vi "IIR Cascade Filter with I.C. PtByPt.vi"(0 "x":dbl format="%0.2f", 1 "IIR Filter Cluster":T1, 3 "Initial Condition":dbl[](array[numeric]), 4 "initialize":bool) -> (5 "Filtered x":dbl format="%0.2f", 6 "Final Condition":dbl[](array[numeric]), 7 "error":i32)   [LabVIEW 2020, in "NI_PtbyPt.lvlib"]
doc: "Filters <B>x</B> using the cascade form of the IIR filter specified by the <B>IIR Filter Cluster</B>."
uses:
  <vilib>/ptbypt/NI_PtbyPt.lvlib
  <vilib>/Analysis/baseanly.llb/IIR Cascade Filter (DBL).vi
  <vilib>/Analysis/NI_AALBase.lvlib
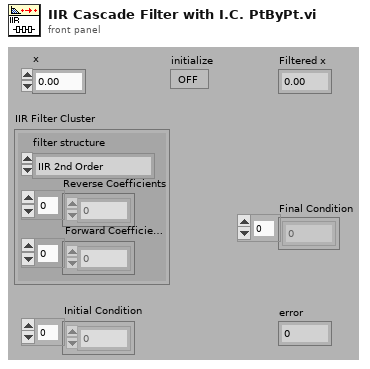
[diagram p1: front panel]
types:
  T1 = cluster{"filter structure":enum32{"IIR 2nd Order", "IIR 4th Order"}, "Reverse Coefficients":dbl[], "Forward Coefficients":dbl[]}
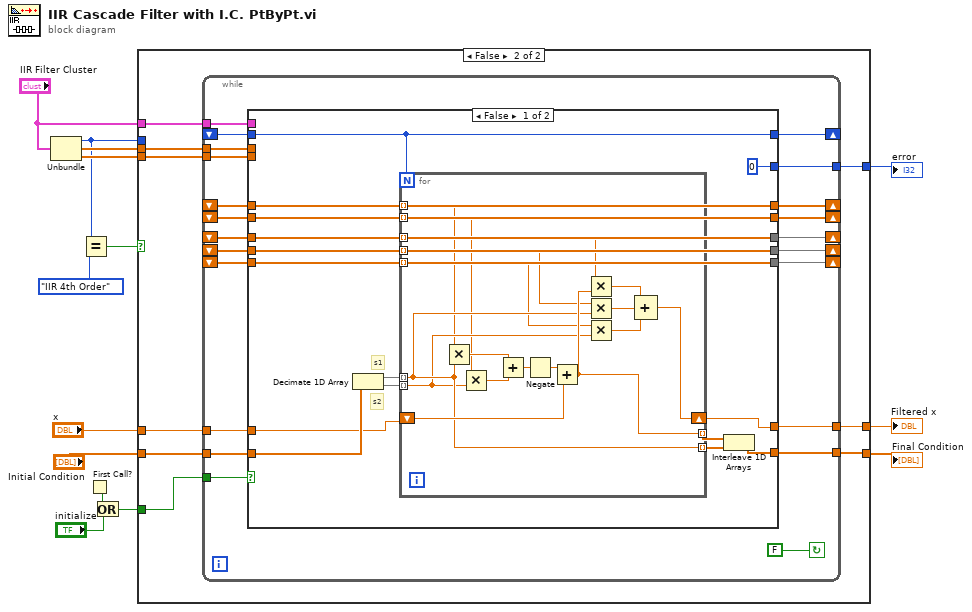
[diagram p0: block diagram]
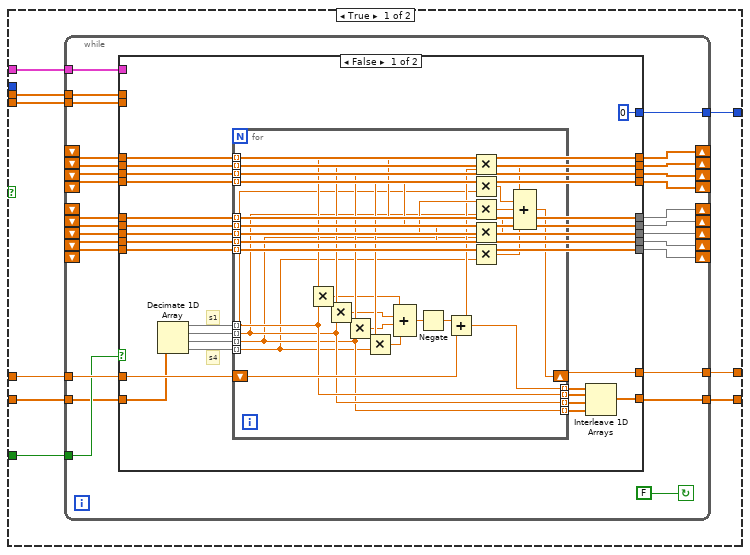
[diagram p2: hidden frame]
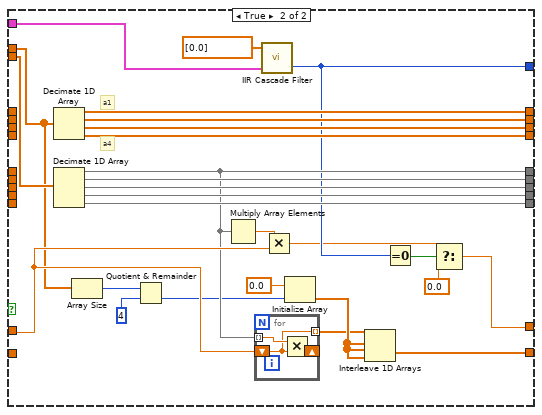
[diagram p3: hidden frame]
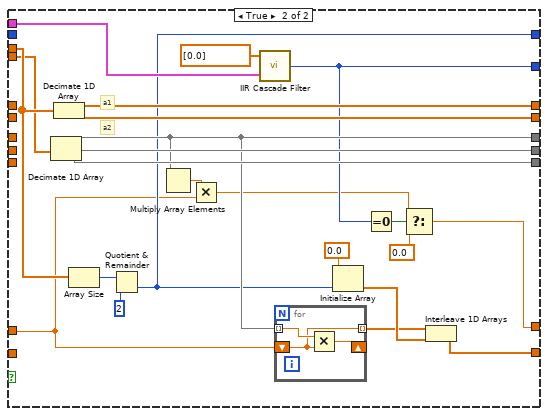
[diagram p4: hidden frame]
diagram:
  n1 = Unbundle("IIR Filter Cluster") -> ("filter structure"=w11:enum32{"IIR 2nd Order", "IIR 4th Order"}, "Reverse Coefficients"=w12:dbl[], "Forward Coefficients"=w13:dbl[])
  n2 = Equal?(x=w11, y=enum32{"IIR 2nd Order", "IIR 4th Order"}."IIR 4th Order") -> (x = y?=w9:bool)
  n3 = First Call?() -> (First Call?: T/F=w6:bool)
  n4 = Or(x=w6, y="initialize") -> (x .or. y?=w7:bool)
  n5 = case shown="False" w9 {
    tunnel: "x" -> [w22 w138]
    tunnel: w13 -> [w20 w136]
    tunnel: w11 -> [_ _]
    tunnel: w12 -> [w21 w137]
    tunnel: [w19 w135] -> w8
    tunnel: w7 -> [w23 w139]
    tunnel: "IIR Filter Cluster" -> [w18 w134]
    tunnel: [w17 w133] -> w4
    tunnel: "Initial Condition" -> [w15 w131]
    tunnel: [w16 w132] -> w2
    frame True {
      n6 = while {
        tunnel: w15 -> [w24]
        tunnel: [w25] -> w16
        tunnel: [w27] -> w17
        tunnel: w18 -> [w28]
        tunnel: [w30] -> w19
        shift-left: _ -> [w31]
        shift-right: [w32] -> _
        shift-left: _ -> [w33]
        shift-right: [w35] -> _
        shift-left: _ -> [w34]
        shift-right: [w36] -> _
        shift-left: _ -> [w37]
        shift-right: [w38] -> _
        tunnel: w22 -> [w39]
        tunnel: w21 -> [w40]
        shift-left: _ -> [w41]
        shift-right: [w43] -> _
        shift-left: _ -> [w42]
        shift-right: [w44] -> _
        shift-left: _ -> [w46]
        shift-right: [w49] -> _
        shift-left: _ -> [w45]
        shift-right: [w48] -> _
        shift-left: _ -> [w47]
        shift-right: [w50] -> _
        tunnel: w20 -> [w51]
        tunnel: w23 -> [w26]
        stop <- FALSE continue-if-true
        n7 = case shown="False" w26 {
          tunnel: w51 -> [_ w116]
          tunnel: [w68 w123] -> w50
          tunnel: [w67 w122] -> w49
          tunnel: [w66 w121] -> w48
          tunnel: w47 -> [w68 _]
          tunnel: w46 -> [w67 _]
          tunnel: w45 -> [w66 _]
          tunnel: [w71 w125] -> w44
          tunnel: [w70 w124] -> w43
          tunnel: w42 -> [w71 _]
          tunnel: w41 -> [w70 _]
          tunnel: w40 -> [_ w104]
          tunnel: w39 -> [w60 w114]
          tunnel: [w72 w126] -> w38
          tunnel: w37 -> [w72 _]
          tunnel: [w69 w113] -> w36
          tunnel: [w65 w120] -> w35
          tunnel: w34 -> [w69 _]
          tunnel: w33 -> [w65 _]
          tunnel: [w73 w127] -> w32
          tunnel: w31 -> [w73 _]
          tunnel: [w58 w106] -> w30
          tunnel: w24 -> [w59 _]
          tunnel: [w53 w115] -> w25
          tunnel: w28 -> [_ w111]
          tunnel: [0 ("error") w109] -> w27
          frame False {
            # "s4"
            # "s1"
            n8 = Decimate 1D Array(w59) -> (w64:dbl[], w63:dbl[], w62:dbl[], w61:dbl[])
            n9 = for {
              tunnel: w71 -> [w98] mode=indexing
              tunnel: w70 -> [w97] mode=indexing
              tunnel: w68 -> [w89] mode=indexing
              tunnel: w67 -> [w88] mode=indexing
              tunnel: w66 -> [w87] mode=indexing
              tunnel: w72 -> [w99] mode=indexing
              tunnel: w65 -> [w86] mode=indexing
              tunnel: w73 -> [w100] mode=indexing
              tunnel: w69 -> [w90] mode=indexing
              tunnel: w64 -> [w77] mode=indexing
              tunnel: w63 -> [w76] mode=indexing
              tunnel: w62 -> [w75] mode=indexing
              tunnel: w61 -> [w74] mode=indexing
              tunnel: [w78] -> w57 mode=indexing
              tunnel: [w75] -> w54 mode=indexing
              tunnel: [w76] -> w55 mode=indexing
              tunnel: [w77] -> w56 mode=indexing
              shift-right: [w79] -> w58
              shift-left: w60 -> [w80]
              n10 = Multiply(x=w100, y=w77) -> (x*y=w96:dbl)
              n11 = Multiply(x=w99, y=w76) -> (x*y=w95:dbl)
              n12 = Multiply(x=w98, y=w75) -> (x*y=w94:dbl)
              n13 = Multiply(x=w97, y=w74) -> (x*y=w93:dbl)
              n14 = Compound Arithmetic op=ADD(w96, w95, w94, w93) -> (w92:dbl)
              n15 = Negate(x=w92) -> (-x=w91:dbl)
              n16 = Add(x=w91, y=w80) -> (x+y=w78:dbl)
              n17 = Multiply(x=w90, y=w78) -> (x*y=w85:dbl)
              n18 = Multiply(x=w89, y=w77) -> (x*y=w84:dbl)
              n19 = Multiply(x=w88, y=w76) -> (x*y=w83:dbl)
              n20 = Multiply(x=w87, y=w75) -> (x*y=w82:dbl)
              n21 = Multiply(x=w86, y=w74) -> (x*y=w81:dbl)
              n22 = Compound Arithmetic op=ADD(w85, w84, w83, w82, w81) -> (w79:dbl)
            }
            n23 = Interleave 1D Arrays(w57, w56, w55, w54) -> (w53:dbl[])
          }
          frame True {
            # "a4"
            # "a1"
            n24 = Decimate 1D Array(w104) -> (w127:dbl[], w126:dbl[], w125:dbl[], w124:dbl[])
            n25 = Decimate 1D Array(w116) -> (w113:dbl[], w123:dbl[], w122:dbl[], w121:dbl[], w120:dbl[])
            n26 = Array Size(array=w104) -> (size(s)=w103:i32)
            n27 = Quotient & Remainder(x=w103, y=4) -> (floor(x/y)=w101:i32)  [unwired: 1 out]
            n28 = Multiply Array Elements(1:w113) -> (0:w119:dbl)
            n29 = for {
              shift-right: [w129] -> _
              shift-left: w114 -> [w128]
              tunnel: w113 -> [w130] mode=indexing
              tunnel: [w128] -> w112 mode=indexing
              n30 = Multiply(x=w130, y=w128) -> (x*y=w129:dbl)
            }
            n31 = call-poly <vilib>:"IIR Cascade Filter.vi"("IIR Filter Cluster"=w111, "X"=dbl[] [0.0]) -> ("error"=w109:i32)  [unwired: 1 in, 1 out]
            n32 = Multiply(x=w119, y=w114) -> (x*y=w107:dbl)
            n33 = Initialize Array(0.0 ("Element Data"), w101) -> (w117:dbl[])
            n34 = Interleave 1D Arrays(w112, w117, w117, w117) -> (w115:dbl[])
            n35 = Equal To 0?(x=w109) -> (x = 0?=w108:bool)
            n36 = Select(t=w107, s=w108, f=0.0) -> (s? t:f=w106:dbl)
          }
        }
      }
    }
    frame False {
      n37 = while {
        tunnel: w131 -> [w140]
        tunnel: [w141] -> w132
        tunnel: [w143] -> w133
        tunnel: w134 -> [w144]
        tunnel: [w146] -> w135
        shift-left: _ -> [w149]
        shift-right: [w150] -> _
        shift-left: _ -> [w151]
        shift-right: [w152] -> _
        shift-left: _ -> [w153]
        shift-right: [w154] -> _
        tunnel: w138 -> [w155]
        tunnel: w137 -> [w156]
        shift-left: _ -> [w157]
        shift-right: [w159] -> _
        shift-left: _ -> [w158]
        shift-right: [w160] -> _
        shift-left: _ -> [w147]
        shift-right: [w148] -> _
        tunnel: w136 -> [w161]
        tunnel: w139 -> [w142]
        stop <- FALSE continue-if-true
        n38 = case shown="False" w142 {
          tunnel: w161 -> [_ w200]
          tunnel: [w173 w214] -> w160
          tunnel: [w172 w213] -> w159
          tunnel: w158 -> [w173 _]
          tunnel: w157 -> [w172 _]
          tunnel: w156 -> [_ w208]
          tunnel: w155 -> [w163 w199]
          tunnel: [w170 w215] -> w154
          tunnel: w153 -> [w170 _]
          tunnel: [w174 w206] -> w152
          tunnel: w151 -> [w174 _]
          tunnel: [w171 w216] -> w150
          tunnel: w149 -> [w171 _]
          tunnel: [w175 w202] -> w148
          tunnel: w147 -> [w175 _]
          tunnel: [w164 w194] -> w146
          tunnel: w140 -> [w176 _]
          tunnel: [w165 w209] -> w141
          tunnel: w144 -> [_ w204]
          tunnel: [0 ("error") w198] -> w143
          frame False {
            # "s2"
            # "s1"
            n39 = Decimate 1D Array(w176) -> (w169:dbl[], w168:dbl[])
            n40 = for {
              N: w175 -> [_]
              tunnel: w169 -> [w183] mode=indexing
              tunnel: w168 -> [w182] mode=indexing
              tunnel: [w184] -> w167 mode=indexing
              tunnel: [w183] -> w166 mode=indexing
              shift-right: [w185] -> w164
              shift-left: w163 -> [w186]
              tunnel: w174 -> [w181] mode=indexing
              tunnel: w173 -> [w180] mode=indexing
              tunnel: w172 -> [w179] mode=indexing
              tunnel: w171 -> [w178] mode=indexing
              tunnel: w170 -> [w177] mode=indexing
              n41 = Multiply(x=w178, y=w183) -> (x*y=w193:dbl)
              n42 = Multiply(x=w177, y=w182) -> (x*y=w192:dbl)
              n43 = Add(x=w193, y=w192) -> (x+y=w191:dbl)
              n44 = Negate(x=w191) -> (-x=w190:dbl)
              n45 = Add(x=w190, y=w186) -> (x+y=w184:dbl)
              n46 = Multiply(x=w181, y=w184) -> (x*y=w189:dbl)
              n47 = Multiply(x=w180, y=w183) -> (x*y=w188:dbl)
              n48 = Multiply(x=w179, y=w182) -> (x*y=w187:dbl)
              n49 = Compound Arithmetic op=ADD(w189, w188, w187) -> (w185:dbl)
            }
            n50 = Interleave 1D Arrays(w167, w166) -> (w165:dbl[])
          }
          frame True {
            # "a2"
            # "a1"
            n51 = Decimate 1D Array(w200) -> (w206:dbl[], w214:dbl[], w213:dbl[])
            n52 = Decimate 1D Array(w208) -> (w216:dbl[], w215:dbl[])
            n53 = Array Size(array=w208) -> (size(s)=w201:i32)
            n54 = Quotient & Remainder(x=w201, y=2) -> (floor(x/y)=w202:i32)  [unwired: 1 out]
            n55 = Multiply Array Elements(1:w206) -> (0:w212:dbl)
            n56 = Multiply(x=w212, y=w199) -> (x*y=w196:dbl)
            n57 = call-poly <vilib>:"IIR Cascade Filter.vi"("IIR Filter Cluster"=w204, "X"=dbl[] [0.0]) -> ("error"=w198:i32)  [unwired: 1 in, 1 out]
            n58 = for {
              shift-right: [w218] -> _
              shift-left: w199 -> [w217]
              tunnel: w206 -> [w219] mode=indexing
              tunnel: [w217] -> w205 mode=indexing
              n59 = Multiply(x=w219, y=w217) -> (x*y=w218:dbl)
            }
            n60 = Initialize Array(0.0 ("Element Data"), w202) -> (w207:dbl[])
            n61 = Equal To 0?(x=w198) -> (x = 0?=w197:bool)
            n62 = Select(t=w196, s=w197, f=0.0) -> (s? t:f=w194:dbl)
            n63 = Interleave 1D Arrays(w205, w207) -> (w209:dbl[])
          }
        }
      }
    }
  }
  "Filtered x" <- w8
  "error" <- w4
  "Final Condition" <- w2
